vi "create_LSID.vi"(8 "error in (no error)":errorcluster, 10 "namespace":string) -> (0 "error out":errorcluster, 2 "LSID":string)   [LabVIEW 2010]
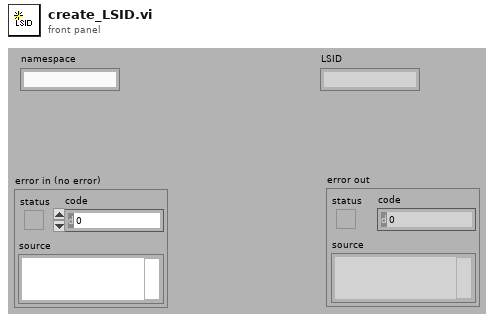
[diagram p1: front panel]
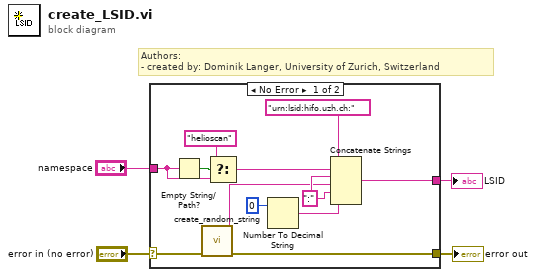
[diagram p0: block diagram]
diagram:
  # "Authors: \n- created by: Dominik Langer, University of Zurich, Switzerland"
  n1 = case shown="No Error" "error in (no error)" {
    selector: "error in (no error)" -> [w9 w17]
    tunnel: [w8 w17] -> w3
    tunnel: "namespace" -> [w5 _]
    tunnel: [w6 _] -> w1
    frame No Error {
      w14 = ":"
      n2 = Empty String/Path?(string/path=w5) -> (empty?=w7:bool)
      n3 = call "create_random_string.vi"("error in (no error)"=w9) -> ("error out"=w8:errorcluster, "random string"=w10:string)  [unwired: 9 in]
      n4 = Select(t="helioscan", s=w7, f=w5) -> (s? t:f=w12:string)
      n5 = Number To Decimal String(number=0) -> (decimal integer string=w16:string)  [unwired: 1 in]
      n6 = Concatenate Strings("urn:lsid:hifo.uzh.ch:" ("string"), w12, w14, w10, w14, w16) -> (w6:string)
    }
    frame Error {
    }
  }
  "LSID" <- w1
  "error out" <- w3
